vi "Test Case, Is Terminate.vi"() -> ()   [LabVIEW 2010]
panel:
  in  "code (-1)":i32=-1
  out "terminated":bool
  in  "stop":bool
  out "error out":errorcluster
  in  "error in":errorcluster
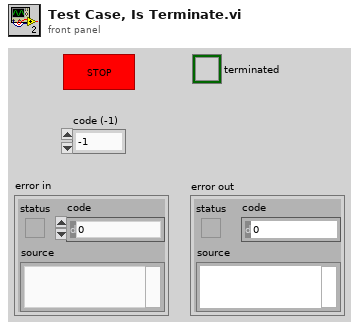
[diagram p1: front panel]
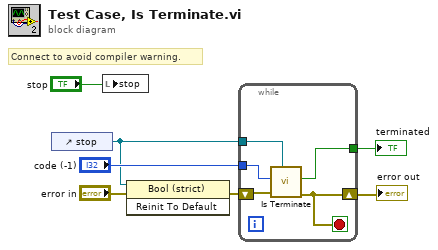
[diagram p0: block diagram]
diagram:
  # "Connect to avoid compiler warning."
  n1 = control-ref of="stop"() -> (w4:refnum<vi>)
  n2 = local write "stop"("stop") -> ()
  n3 = invoke class="Bool (strict)" method="Reinit To Default"(reference=w4, error in="error in") -> (error out=w2:errorcluster)  [unwired: 1 in, 2 out]
  n4 = while {
    tunnel: w4 -> [w11]
    shift-right: [w10] -> w7
    shift-left: w2 -> [w12]
    tunnel: [w9] -> w6
    tunnel: "code (-1)" -> [w8]
    stop <- w10 stop-if-true
    n5 = call "Is Terminate.vi"("Stop Refnum"=w11, "error in"=w12, "code (-1)"=w8) -> ("error out"=w10:errorcluster, "terminated"=w9:bool)  [unwired: 5 in]
  }
  "error out" <- w7
  "terminated" <- w6
